vi "XMLGetCells.vi"(11 "XML":string) -> (3 "Cells":string[](array[string]))   [LabVIEW 2014]
uses:
  <vilib>/regexp/Match Regular Expression.xnode
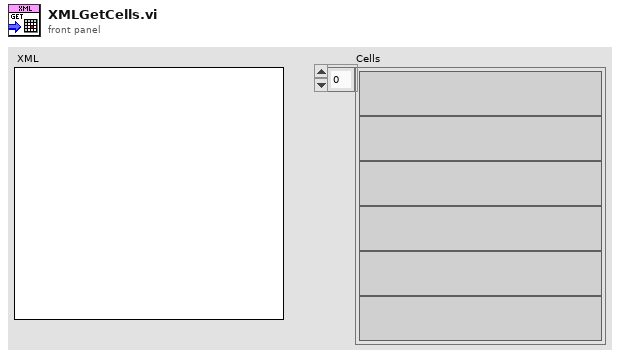
[diagram p1: front panel]
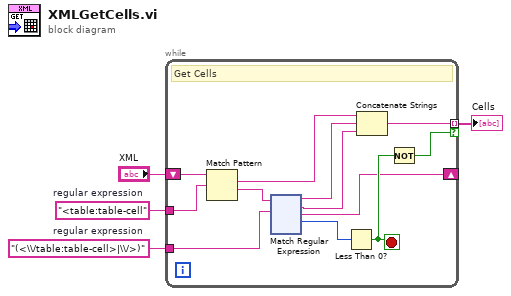
[diagram p0: block diagram]
diagram:
  w2 = "(<\\/table:table-cell>|\\/>)"  # regular expression
  w1 = "<table:table-cell"  # regular expression
  n1 = while {
    shift-right: [w6] -> _
    shift-left: "XML" -> [w16]
    tunnel: w1 -> [w15]
    tunnel: w2 -> [w9]
    tunnel: [w13] -> w3 mode=indexing if=w11
    stop <- w12 stop-if-true
    # "Get Cells"
    n2 = Match Pattern(string=w16, regular expression=w15) -> (match substring=w14:string, after substring=w10:string)  [unwired: 1 in, 2 out]
    n3 = xnode "Match Regular Expression"("input string"=w10, "regular expression"=w9) -> ("before match"=w8:string, "whole match"=w7:string, "after match"=w6:string, "offset past match"=w5:i32)  [unwired: 4 in, 1 out]
    n4 = Less Than 0?(x=w5) -> (x < 0?=w12:bool)
    n5 = Concatenate Strings(w14, w8, w7) -> (w13:string)
    n6 = Not(x=w12) -> (.not. x?=w11:bool)
  }
  "Cells" <- w3
